vi "IPI_Cal_UL.vi"(8 "Result":string="15", 9 "LSL":string, 10 "USL":string, 11 "Standard Value":string) -> (0 "DownLimit":dbl, 1 "LSL":string, 2 "USL":string, 3 "UPLimit":dbl, 4 "passorfali":string)   [LabVIEW 2015]
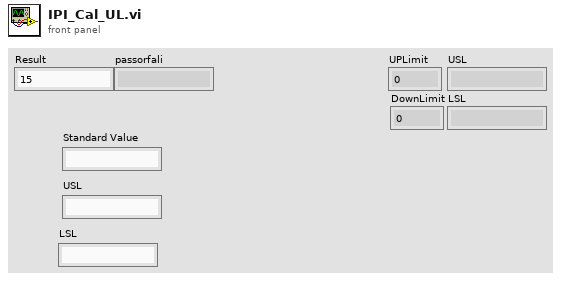
[diagram p1: front panel]
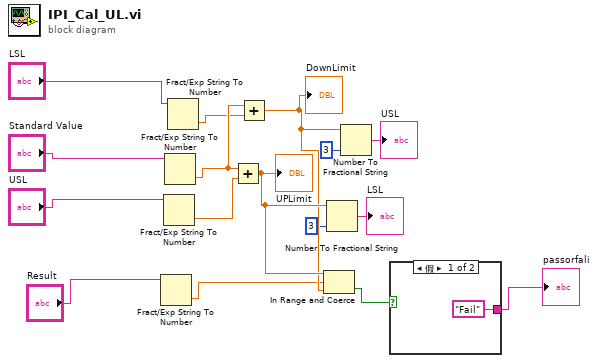
[diagram p0: block diagram]
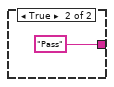
[diagram p2: hidden frame]
diagram:
  n1 = Fract/Exp String To Number(string="Result") -> (number=w5:dbl)  [unwired: 3 in, 1 out]
  n2 = Fract/Exp String To Number(string="USL") -> (number=w13:dbl)  [unwired: 3 in, 1 out]
  n3 = Fract/Exp String To Number(string="Standard Value") -> (number=w12:dbl)  [unwired: 3 in, 1 out]
  n4 = Fract/Exp String To Number(string="LSL") -> (number=w11:dbl)  [unwired: 3 in, 1 out]
  n5 = Add(x=w12, y=w13) -> (x+y=w8:dbl)
  "UPLimit" <- w8
  n6 = Add(x=w12, y=w11) -> (x+y=w7:dbl)
  "DownLimit" <- w7
  n7 = In Range and Coerce(upper limit=w8, x=w5, lower limit=w7) -> (In Range?=w4:bool)  [unwired: 1 out]
  n8 = Number To Fractional String(number=w8, precision (6)=i16 3 ("精度(6)")) -> (F-format string=→"LSL":string)  [unwired: 2 in]
  n9 = Number To Fractional String(number=w7, precision (6)=i16 3 ("精度(6)")) -> (F-format string=→"USL":string)  [unwired: 2 in]
  n10 = case shown="假" w4 {
    tunnel: ["Fail" "Pass"] -> w3
    frame False {
    }
    frame True {
    }
  }
  "passorfali" <- w3
